vi "LEP_RV_LaunchDebug.vi"(8 "error in (no error)":errorcluster) -> (0 "error out":errorcluster)   [LabVIEW 2011]
doc: "Download and execute built VxWorks downloadable module and attach the LabVIEW Embedded debuger."
uses:
  <vilib>/LabVIEW Targets/TargetShared/nitargetDataType.ctl
  LEP_RV_LaunchGlobals.vi
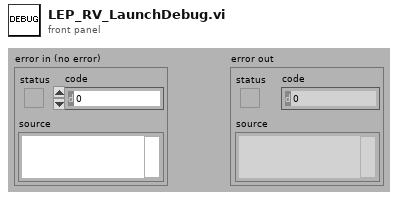
[diagram p1: front panel]
types:
  T1 = typedef "LEP_RV_Config.ctl" = cluster{"Enable debugging":bool, "Debug Options":u16, "Use stack variables":bool, "Generate serial only":bool, "Generate guard code":bool, "Generate Integer Only":bool, "Generate C Function Calls":bool, "ExpressionFolding":bool, "Constant Allocation":u16, "Constant Deallocation":u16, "Build Specification ID":string, "Preprocessor symbols (define)":string, "Compiler Flags":string, "Linker Flags":string, "Mode":u16, "Optimization":u16, "Optimize for time":bool, "Enable cross-module optimization":bool, "Include paths":path[], "Optimize heap size":bool, "Use MicroLib":bool, "Debug Mode":u16, "Enable profile information":bool, "Host name":string, "Use DHCP":bool, "IP address":string, "Subnet mask":string, "Gateway":string, "Primary DNS":string, "Secondary DNS":string, "MAC in target memory":bool, "MAC address":string, "Console output":u16, "Target serial port":u16}
  T2 = typedef "nitargetDataType.ctl" = cluster{"enable array":bool, "enable cluster":bool, "write sub VI ctrl enable":bool}
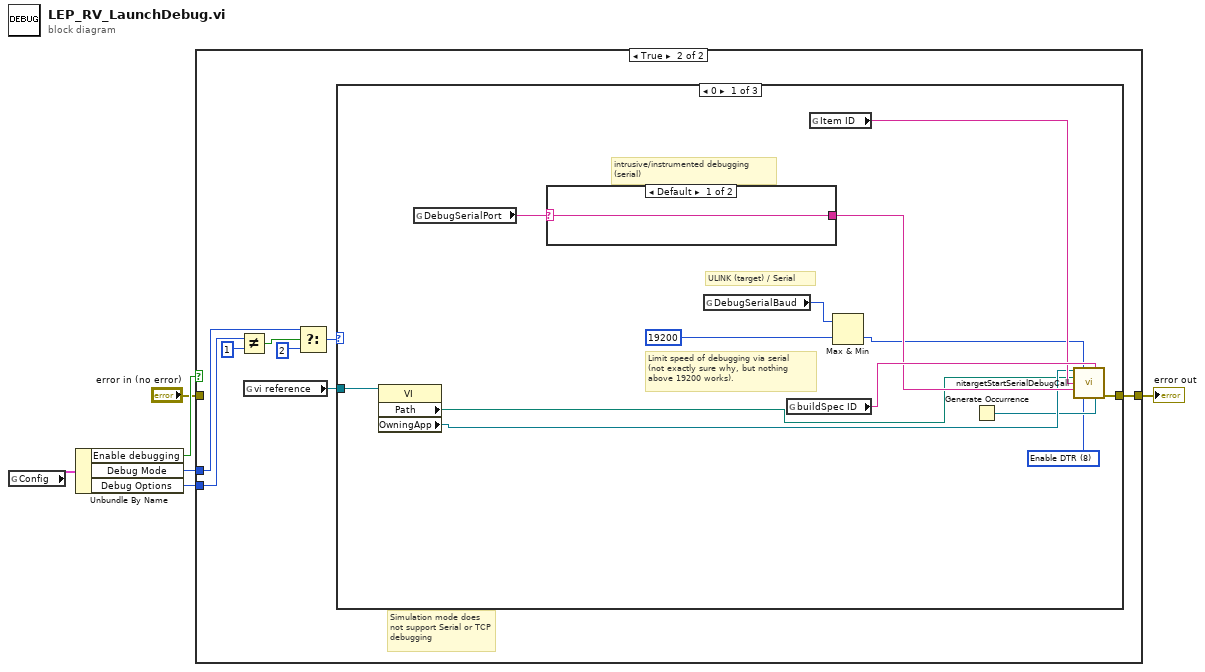
[diagram p0: block diagram]
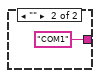
[diagram p3: hidden frame]
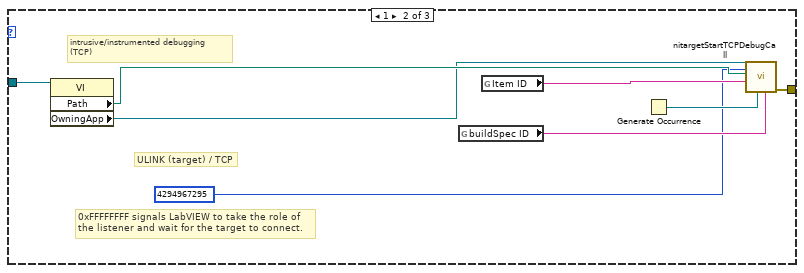
[diagram p4: hidden frame]
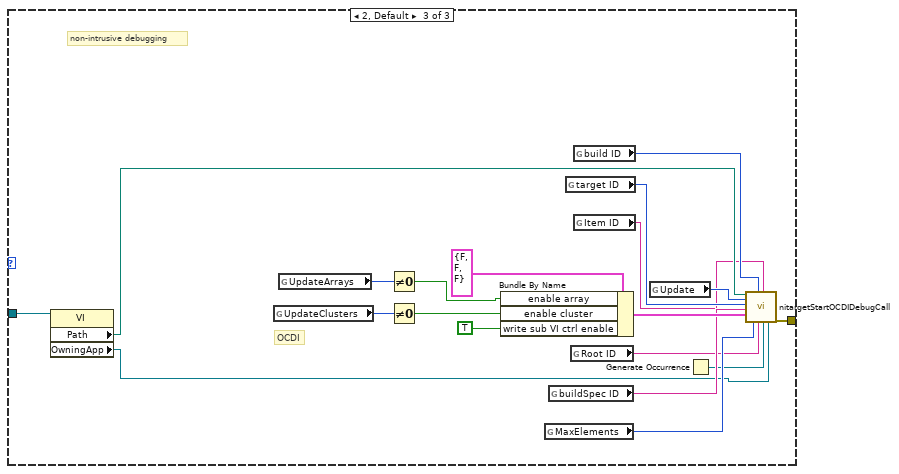
[diagram p5: hidden frame]
diagram:
  n1 = global read "LEP_RV_LaunchGlobals.vi" "Config"() -> (w2:T1)
  n2 = Unbundle By Name(w2) -> ("Enable debugging"=w5:bool, "Debug Mode"=w4:u16, "Debug Options"=w3:u16)
  n3 = case shown="True" w5 {
    tunnel: [w7 w9] -> w6
    tunnel: w4 -> [_ w11]
    tunnel: w3 -> [_ w15]
    tunnel: "error in (no error)" -> [w7 _]
    frame False {
      # "No debugging enabled"
    }
    frame True {
      # "Simulation mode does not support Serial or TCP debugging"
      n4 = Not Equal?(x=w15, y=u16 1) -> (x != y?=w10:bool)
      n5 = global read "LEP_RV_LaunchGlobals.vi" "vi reference"() -> (w8:refnum<vi>)
      n6 = Select(t=w11, s=w10, f=u16 2 ("Debug Mode")) -> (s? t:f=w13:u16)
      n7 = case shown="0" w13 {
        tunnel: [w25 w38 w51] -> w9
        tunnel: w8 -> [w24 w37 w48]
        frame 0 {
          w16 = u16 8 items=["None"=0, "XON/XOFF"=1, "RTS/CTS"=2, "XON/XOFF & RTS/CTS"=3, "DTR/DSR"=4, "XON/XOFF & DTR/DSR"=5, "Enable DTR"=8] ("flow control")
          # "Limit speed of debugging via serial\n(not exactly sure why, but nothing\nabove 19200 works)."
          # "ULINK (target) / Serial"
          # "intrusive/instrumented debugging\n(serial)"
          n8 = property class="VI"(reference=w24) -> ("Path"=w18:path, "OwningApp"=w19:refnum<vi>)  [unwired: 1 in, 2 out]
          n9 = global read "LEP_RV_LaunchGlobals.vi" "DebugSerialPort"() -> (w27:string)
          n10 = case shown="Default" w27 {
            selector: w27 -> [w29 _]
            tunnel: [w29 "COM1" ("t")] -> w21
            frame Default {
            }
            frame "" {
            }
          }
          n11 = global read "LEP_RV_LaunchGlobals.vi" "DebugSerialBaud"() -> (w26:u32)
          n12 = global read "LEP_RV_LaunchGlobals.vi" "buildSpec ID"() -> (w23:string)
          n13 = global read "LEP_RV_LaunchGlobals.vi" "Item ID"() -> (w22:string)
          n14 = Max & Min(x=w26, y=u32 19200) -> (min(x,y)=w20:u32)  [unwired: 1 out]
          n15 = Generate Occurrence() -> (w17:refnum<k4>)
          n16 = call <vilib>:"nitargetStartSerialDebugCall.vi"("context"=w19, "baud rate"=w20, "buildSpec ID"=w23, "vi path"=w18, "item ID"=w22, "serial port"=w21, "flow control"=w16, "occurrence"=w17) -> ("error out"=w25:errorcluster)  [unwired: 7 in]
        }
        frame 1 {
          # "0xFFFFFFFF signals LabVIEW to take the role of the listener and wait for the target to connect."
          # "ULINK (target) / TCP"
          # "intrusive/instrumented debugging\n(TCP)"
          n17 = property class="VI"(reference=w37) -> ("Path"=w36:path, "OwningApp"=w35:refnum<vi>)  [unwired: 1 in, 2 out]
          n18 = global read "LEP_RV_LaunchGlobals.vi" "buildSpec ID"() -> (w32:string)
          n19 = global read "LEP_RV_LaunchGlobals.vi" "Item ID"() -> (w33:string)
          n20 = Generate Occurrence() -> (w34:refnum<k4>)
          n21 = call <vilib>:"nitargetStartTCPDebugCall.vi"("buildSpec ID"=w32, "occurrence"=w34, "ipAddress"=u32 4294967295, "item ID"=w33, "vi path"=w36, "context"=w35) -> ("error out"=w38:errorcluster)  [unwired: 5 in]
        }
        frame 2, Default {
          # "non-intrusive debugging"
          # "OCDI"
          n22 = property class="VI"(reference=w48) -> ("Path"=w47:path, "OwningApp"=w39:refnum<vi>)  [unwired: 1 in, 2 out]
          n23 = global read "LEP_RV_LaunchGlobals.vi" "UpdateClusters"() -> (w52:u32)
          n24 = global read "LEP_RV_LaunchGlobals.vi" "UpdateArrays"() -> (w53:u32)
          n25 = Not Equal To 0?(x=w53) -> (x != 0?=w56:bool)
          n26 = Not Equal To 0?(x=w52) -> (x != 0?=w55:bool)
          n27 = Bundle By Name(cluster=T2 {"enable array"=FALSE, "enable cluster"=FALSE, "write sub VI ctrl enable"=FALSE} ("data type"), "enable array"=w56, "enable cluster"=w55, "write sub VI ctrl enable"=TRUE) -> (w50:T2)
          n28 = global read "LEP_RV_LaunchGlobals.vi" "MaxElements"() -> (w49:u32)
          n29 = global read "LEP_RV_LaunchGlobals.vi" "buildSpec ID"() -> (w44:string)
          n30 = global read "LEP_RV_LaunchGlobals.vi" "target ID"() -> (w45:u32)
          n31 = global read "LEP_RV_LaunchGlobals.vi" "Root ID"() -> (w41:string)
          n32 = global read "LEP_RV_LaunchGlobals.vi" "build ID"() -> (w43:u32)
          n33 = global read "LEP_RV_LaunchGlobals.vi" "Item ID"() -> (w42:string)
          n34 = global read "LEP_RV_LaunchGlobals.vi" "Update"() -> (w46:u32)
          n35 = Generate Occurrence() -> (w40:refnum<k4>)
          n36 = call <vilib>:"nitargetStartOCDIDebugCall.vi"("vi path"=w47, "update period"=w46, "target ID"=w45, "buildSpec ID"=w44, "data type"=w50, "max elements"=w49, "build ID"=w43, "Root ID"=w41, "Item ID"=w42, "occurrence"=w40, "context"=w39) -> ("error out"=w51:errorcluster)  [unwired: 8 in]
        }
      }
    }
  }
  "error out" <- w6
